vi "Get Port Baud Rate.vi"(8 "error in":errorcluster, 11 "Port Ref":T1 format="%.0x") -> (0 "error out":errorcluster, 2 "Baud Rate":u32, 3 "Port Ref out":T1 format="%.0x")   [LabVIEW 2020, in "Ballard MIL-STD-1553 Scripting.lvlib"]
uses:
  Ballard MIL-STD-1553 Scripting.lvlib
  <vilib>/NI VeriStand/Custom Device API/Custom Device Item Ref.ctl
  Constants.vi
  <vilib>/NI VeriStand/Custom Device API/Get Item Property (U32).vi
  <vilib>/NI VeriStand/Custom Device API/Custom Device API.lvlib
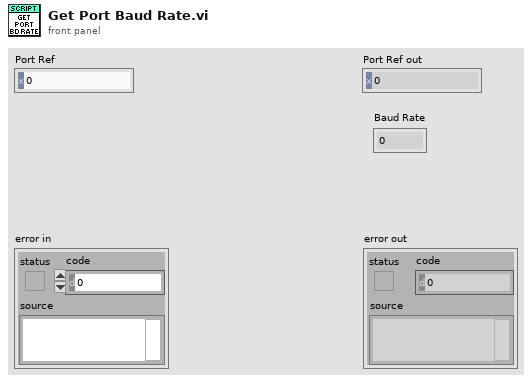
[diagram p1: front panel]
types:
  T1 = typedef "Custom Device API.lvlib/Custom Device Item Ref.ctl" = u64
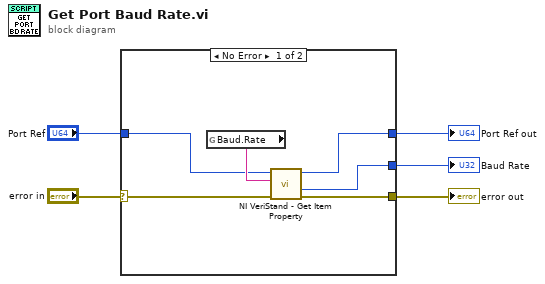
[diagram p0: block diagram]
diagram:
  n1 = case shown="No Error" "error in" {
    selector: "error in" -> [w7 w13]
    tunnel: "Port Ref" -> [w10 w12]
    tunnel: [w9 w13] -> w4
    tunnel: [w8 w12] -> w3
    tunnel: [w6 _] -> w1
    frame No Error {
      n2 = global read "Constants.vi" "Baud.Rate"() -> (w11:string)
      n3 = call-poly <vilib>:"NI VeriStand - Get Item Property.vi"("error in (no error)"=w7, "Property Name"=w11, "Item Ref in"=w10) -> ("error out"=w9:errorcluster, "Value"=w6:u32, "Item Ref out"=w8:T1)  [unwired: 5 in, 1 out]
    }
    frame Error {
    }
  }
  "error out" <- w4
  "Baud Rate" <- w1
  "Port Ref out" <- w3
